vi "BIN_PAQ_year_num_2_filename.vi"(8 "error in":errorcluster, 9 "num":u64, 10 "ext":string, 11 "TableName":string) -> (0 "error out":errorcluster, 2 "FileName":string)   [LabVIEW 2020, in "Sgraph_lib_V1.lvlib" / "DBAL-BIN.lvclass"]
doc: "Binary PAQ file: numeric file identifier to filename\nThis version constructs the YYYY format"
uses:
  DBAL-BIN.lvclass
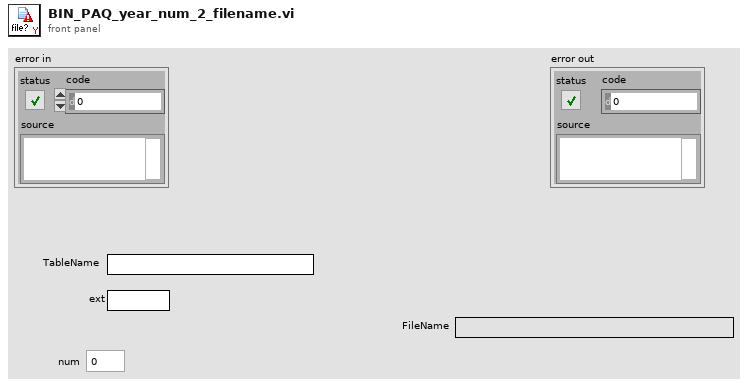
[diagram p1: front panel]
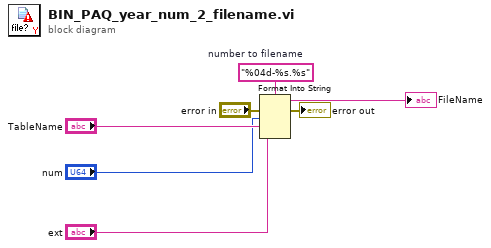
[diagram p0: block diagram]
diagram:
  w7 = "%04d-%s.%s"  # number to filename
  n1 = Format Into String(format string=w7, error in="error in", "num", "TableName", "ext") -> (resulting string=→"FileName":string, error out=→"error out":errorcluster)  [unwired: 1 in]
